vi "2 Tank Filling.vi"() -> ()   [LabVIEW 2021]
panel:
  in  "stop":bool
  in  "OK Button":bool
  out "Tank 1":dbl(slide) scale=0.0..100.0
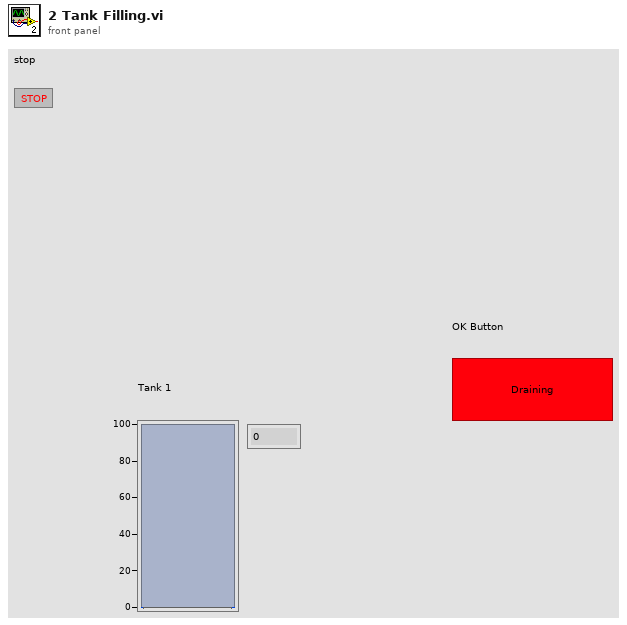
[diagram p1: front panel]
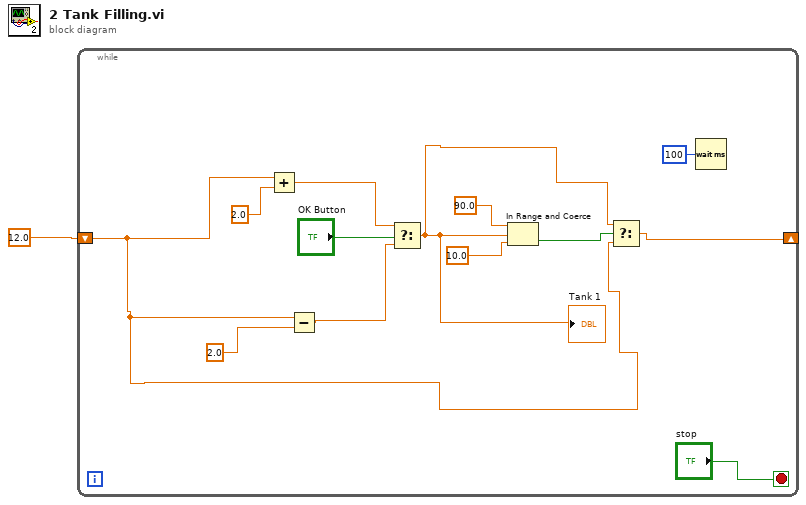
[diagram p0: block diagram]
diagram:
  n1 = while {
    shift-right: [w6] -> _
    shift-left: 12.0 -> [w3]
    stop <- "stop" stop-if-true
    n2 = Add(x=w3, y=2.0) -> (x+y=w11:dbl)
    n3 = Subtract(x=w3, y=2.0) -> (x-y=w10:dbl)
    n4 = Select(t=w11, s="OK Button", f=w10) -> (s? t:f=w4:dbl)
    "Tank 1" <- w4
    n5 = In Range and Coerce(upper limit=90.0, x=w4, lower limit=10.0 ("s? t:f")) -> (In Range?=w7:bool)  [unwired: 1 out]
    n6 = Select(t=w4, s=w7, f=w3) -> (s? t:f=w6:dbl)
    n7 = Wait (ms)(milliseconds to wait=u32 100) -> ()  [unwired: 1 out]
  }
